vi "Init.vi"(8 "error in":errorcluster, 10 "<JSON> Const Action Data":string, 11 "Perform Action Strategy in":refnum<class "Perform Action Strategy.lvclass">) -> (0 "error out":errorcluster, 3 "Perform Action Strategy out":refnum<class "Perform Action Strategy.lvclass">)   [LabVIEW 2023, in "HAL.lvlib" / "Perform Action Strategy.lvclass"]
uses:
  Perform Action Strategy.lvclass
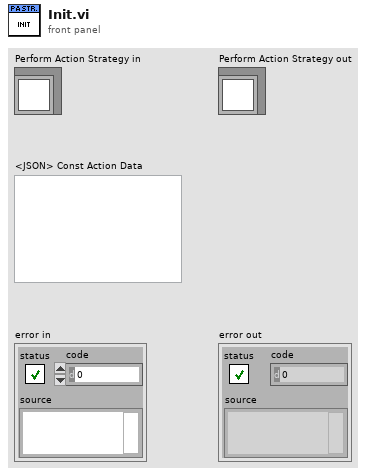
[diagram p1: front panel]
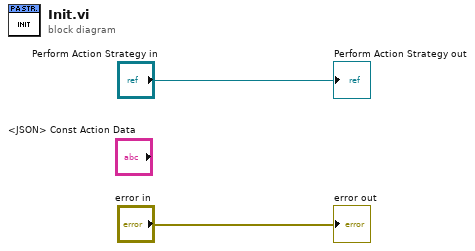
[diagram p0: block diagram]
diagram:
  "error out" <- "error in"
  "Perform Action Strategy out" <- "Perform Action Strategy in"
